vi "FGV_ONOFF.vi"(8 "errin":errorcluster, 10 "CMD":T1, 11 "ONOFF":enum16{"TurnON", "TurnOFF"}(ring)=enum."TurnOFF") -> (0 "errout":errorcluster, 3 "OUT":enum16{"TurnON", "TurnOFF"}(ring))   [LabVIEW 2020]
uses:
  02 SLIM ZEN WS 500/SubVi/FGV.ctl
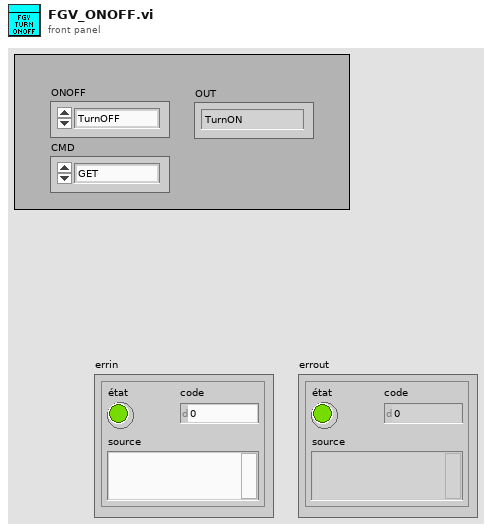
[diagram p1: front panel]
types:
  T1 = typedef "FGV.ctl" = enum16{"GET", "SET", "RAZ"}
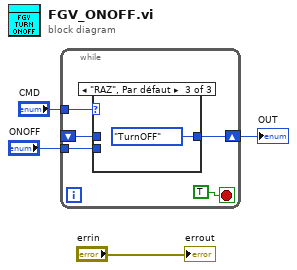
[diagram p0: block diagram]
diagram:
  n1 = while {
    shift-right: [w8] -> w2
    shift-left: _ -> [w7]
    tunnel: "ONOFF" -> [w6]
    tunnel: "CMD" -> [w5]
    stop <- TRUE stop-if-true
    n2 = case shown="\"RAZ\", Par défaut" w5 {
      tunnel: [w10 w11 enum16{"TurnON", "TurnOFF"}."TurnOFF"] -> w8
      tunnel: w7 -> [w10 _ _]
      tunnel: w6 -> [_ w11 _]
      frame "GET" {
      }
      frame "SET" {
      }
      frame "RAZ", Default {
      }
    }
  }
  "OUT" <- w2
  "errout" <- "errin"
